vi "VGD ECL AHMI PF SubVI01.vi"(3 "error in":errorcluster, 4 "Factor diezmado":i32=60, 5 "SUPERIOR":T1, 6 "FRONTAL":T1) -> (0 "error out":errorcluster, 1 "pixmap S":u32[][](array[numeric]), 2 "pixmap F":u32[][](array[numeric]))   [LabVIEW 2020]
uses:
  <vilib>/vision/Image Controls.llb/IMAQ Image.ctl
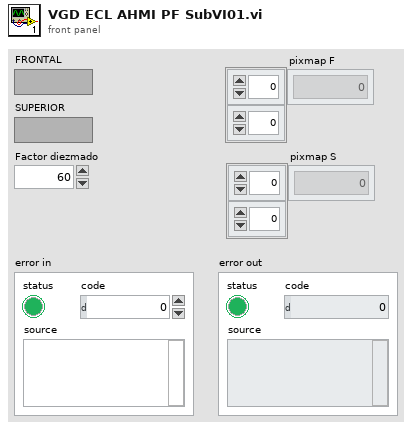
[diagram p1: front panel]
types:
  T1 = typedef "IMAQ Image.ctl" = refnum<image>
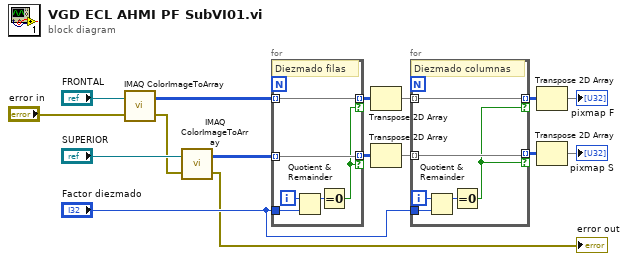
[diagram p0: block diagram]
diagram:
  n1 = call "IMAQ ColorImageToArray"("Image"="FRONTAL", "error in (no error)"="error in") -> ("Image Pixels (U32)"=w14:u32[][], "error out"=w9:errorcluster)  [unwired: 2 in, 1 out]
  n2 = call "IMAQ ColorImageToArray"("Image"="SUPERIOR", "error in (no error)"=w9) -> ("Image Pixels (U32)"=w8:u32[][], "error out"=→"error out":errorcluster)  [unwired: 2 in, 1 out]
  n3 = for {
    tunnel: w14 -> [w22] mode=indexing
    tunnel: [w22] -> w16 mode=indexing if=w17
    tunnel: "Factor diezmado" -> [w19]
    tunnel: w8 -> [w18] mode=indexing
    tunnel: [w18] -> w7 mode=indexing if=w17
    i -> [w21]
    # "Diezmado filas"
    n4 = Quotient & Remainder(x=w21, y=w19) -> (x-y*floor(x/y)=w20:i32)  [unwired: 1 out]
    n5 = Equal To 0?(x=w20) -> (x = 0?=w17:bool)
  }
  n6 = Transpose 2D Array(2D array=w16) -> (transposed array=w15:u32[][])
  n7 = Transpose 2D Array(2D array=w7) -> (transposed array=w6:u32[][])
  n8 = for {
    tunnel: w15 -> [w28] mode=indexing
    tunnel: [w28] -> w12 mode=indexing if=w23
    tunnel: "Factor diezmado" -> [w25]
    tunnel: w6 -> [w24] mode=indexing
    tunnel: [w24] -> w5 mode=indexing if=w23
    i -> [w27]
    # "Diezmado columnas"
    n9 = Quotient & Remainder(x=w27, y=w25) -> (x-y*floor(x/y)=w26:i32)  [unwired: 1 out]
    n10 = Equal To 0?(x=w26) -> (x = 0?=w23:bool)
  }
  n11 = Transpose 2D Array(2D array=w12) -> (transposed array=→"pixmap F":u32[][])
  n12 = Transpose 2D Array(2D array=w5) -> (transposed array=→"pixmap S":u32[][])
